vi "Set State.vi"(8 "error in (no error)":errorcluster, 10 "State":T1, 11 "ATM Controller in":refnum<class "ATM Controller.lvclass">) -> (0 "error out":errorcluster, 3 "ATM Controller out":refnum<class "ATM Controller.lvclass">)   [LabVIEW 2019, in "ATM Controller.lvlib" / "ATM Controller.lvclass"]
uses:
  ATM Controller.lvclass
  State -Enum.ctl
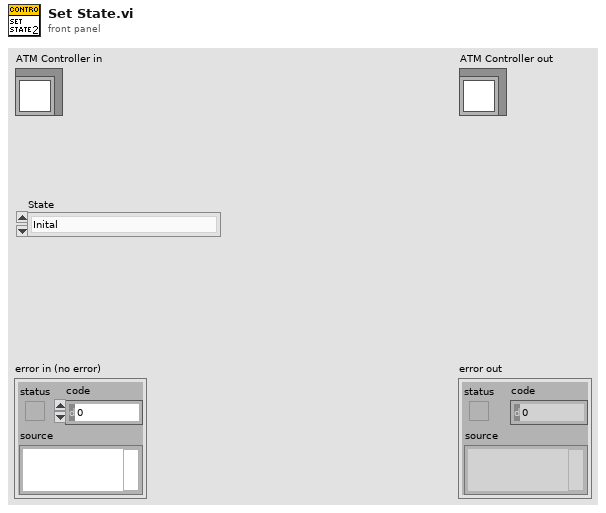
[diagram p1: front panel]
types:
  T1 = typedef "ATM Controller.lvlib/ATM Controller.lvclass/State -Enum.ctl" = enum16{"Inital", "Idle", "Login", "Balance Inquiry", "Deposit", "Withdrawal", "Fast Cash", "Terminate"}
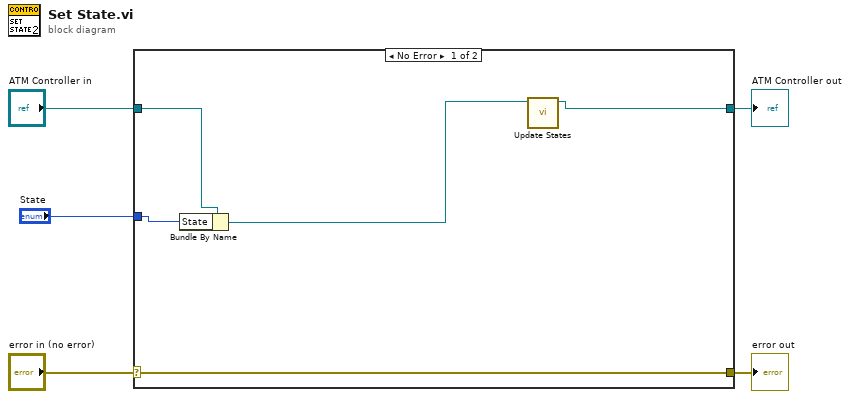
[diagram p0: block diagram]
diagram:
  n1 = case shown="No Error" "error in (no error)" {
    selector: "error in (no error)" -> [w10 w12]
    tunnel: [w10 w12] -> w4
    tunnel: [w6 w11] -> w2
    tunnel: "ATM Controller in" -> [w9 w11]
    tunnel: "State" -> [w8 _]
    frame No Error {
      n2 = Bundle By Name(cluster=w9, "State"=w8) -> (w7:refnum<class "ATM Controller.lvclass">)
      n3 = call "Update States.vi"("ATM Controller in"=w7) -> ("ATM Controller out"=w6:refnum<class "ATM Controller.lvclass">)  [unwired: 9 in, 1 out]
    }
    frame Error {
    }
  }
  "error out" <- w4
  "ATM Controller out" <- w2
